vi "TP.vi"(8 "error in (no error)":errorcluster, 10 "Axis Number":i32, 11 "Agilis in":T1) -> (0 "error out":errorcluster, 2 "Accumulated Steps":i32, 3 "Agilis out":T1)   [LabVIEW 2016, in "Drivers.lvlib" / "Agilis.lvlib"]
doc: "Returns the number of accumulated steps in positive minus negative directions since powering the controller or the last ZP command. \n\nThe step size are not 100% repeatable and vary between postive and negative direction. Furthermore, the step size can be modified using SU. Consequently, TP provides only limited information about the actual position of the device. In particular, device can be at very different positions even though TPs return same results."
uses:
  Agilis.lvlib
  AgilisCmdLib Refnum.ctl
  C:/Users/MyUser/Desktop/Trace Grabber/Drivers/Agilis/AgilisCmdLib.dll
  AgilisCmdLib.dll
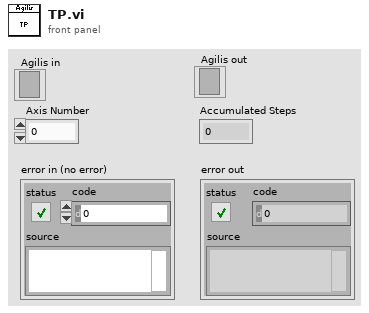
[diagram p1: front panel]
types:
  T1 = typedef "Drivers.lvlib/Agilis.lvlib/AgilisCmdLib Refnum.ctl" = refnum<k24>
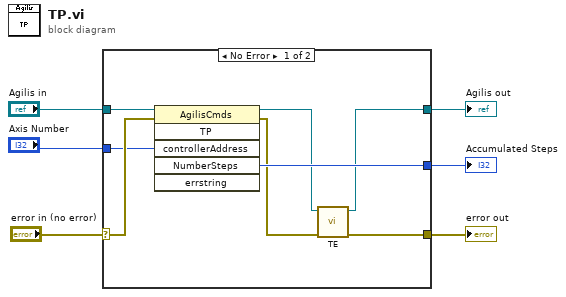
[diagram p0: block diagram]
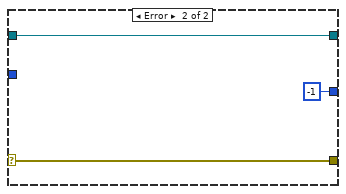
[diagram p2: hidden frame]
diagram:
  n1 = case shown="No Error" "error in (no error)" {
    selector: "error in (no error)" -> [w13 w17]
    tunnel: "Agilis in" -> [w14 w16]
    tunnel: [w7 w16] -> w4
    tunnel: [w9 w17] -> w3
    tunnel: [w11 -1 ("ChannelNumber")] -> w2
    tunnel: "Axis Number" -> [w12 _]
    frame No Error {
      n2 = invoke class="AgilisCmds" method="TP"(reference=w14, error in=w13, "controllerAddress"=w12) -> (reference out=w8:T1, error out=w10:errorcluster, "NumberSteps"=w11:i32)  [unwired: 3 in, 3 out]
      n3 = call "TE.vi"("error in (no error)"=w10, "Agilis in"=w8) -> ("error out"=w9:errorcluster, "Agilis out"=w7:T1)  [unwired: 8 in]
    }
    frame Error {
    }
  }
  "Agilis out" <- w4
  "error out" <- w3
  "Accumulated Steps" <- w2
